vi "Start or Acquire.vi"(6 "Daq cmd":T2, 8 "error in (no error)":errorcluster) -> (0 "error out":errorcluster, 2 "Server Stats":T1={"scan rate"=10.0, "# connections"=0, "channel settings"=[]} {"channel settings"."lower input limits" format="%.4f"; "channel settings"."upper input limits" format="%.4f"; "scan rate" format="%.2f"}, 3 "task out":refnum<k21>)   [LabVIEW 2012]
uses:
  Local Daq Config.ctl
  Daq cmd.ctl
  DataServer/Server stats.ctl
  read-write.ctl
  ini interface.ctl
  <vilib>/DAQmx/read.llb/DAQmx Read (Analog 2D DBL NChan NSamp).vi
  <vilib>/DAQmx/create/channels.llb/DAQmx Create Channel (AI-Voltage-Basic).vi
  <vilib>/DAQmx/configure/timing.llb/DAQmx Timing (Sample Clock).vi
  <vilib>/DAQmx/miscellaneous.llb/DAQmx Fill In Error Info.vi
panel:
  out "data":dbl[][](array[numeric]) format="%0.2f"
  out "Channels":string
  in  "max buffer":i32=100
  out "Local Daq Config":T3={"Sample rate (Hz)"=1.0, "Over sample factor"=1.0, "Terminal Configuration"=enum."Single Ended", "Device"=0, "Max Voltage"=0} {"Device" items=["Dev1"]; "Over sample factor" min=1.0 max=125.0 step=1.0; "Sample rate (Hz)" min=1.0 max=10000.0 step=1.0}
  # "Hz"
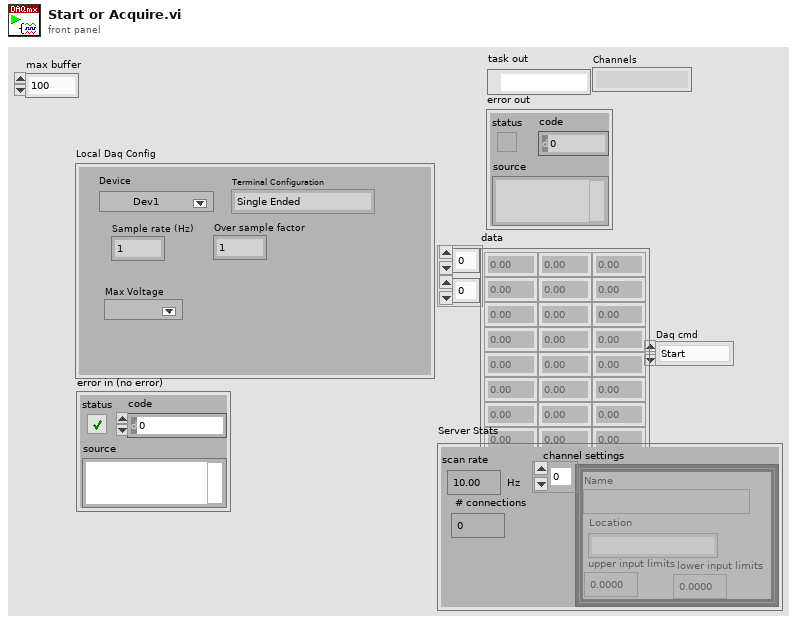
[diagram p1: front panel]
types:
  T1 = typedef "Server stats.ctl" = cluster{"scan rate":dbl, "# connections":i32, "channel settings":cluster{"Name":string, "upper input limits":sgl, "lower input limits":sgl, "Location":string}[]}
  T2 = typedef "Daq cmd.ctl" = enum16{"Start", "Get one scan", "Server Stats", "Stop Acquisition"}
  T3 = typedef "Local Daq Config.ctl" = cluster{"Sample rate (Hz)":dbl, "Over sample factor":dbl, "Terminal Configuration":enum16{"Single Ended", "Differential"}, "Device":u16, "Max Voltage":u16}
  T4 = typedef "ini interface.ctl" = enum16{"dataserver list", "dataserver", "com port", "stamp model", "Local Daq"}
  T5 = typedef "read-write.ctl" = enum16{"read", "write"}
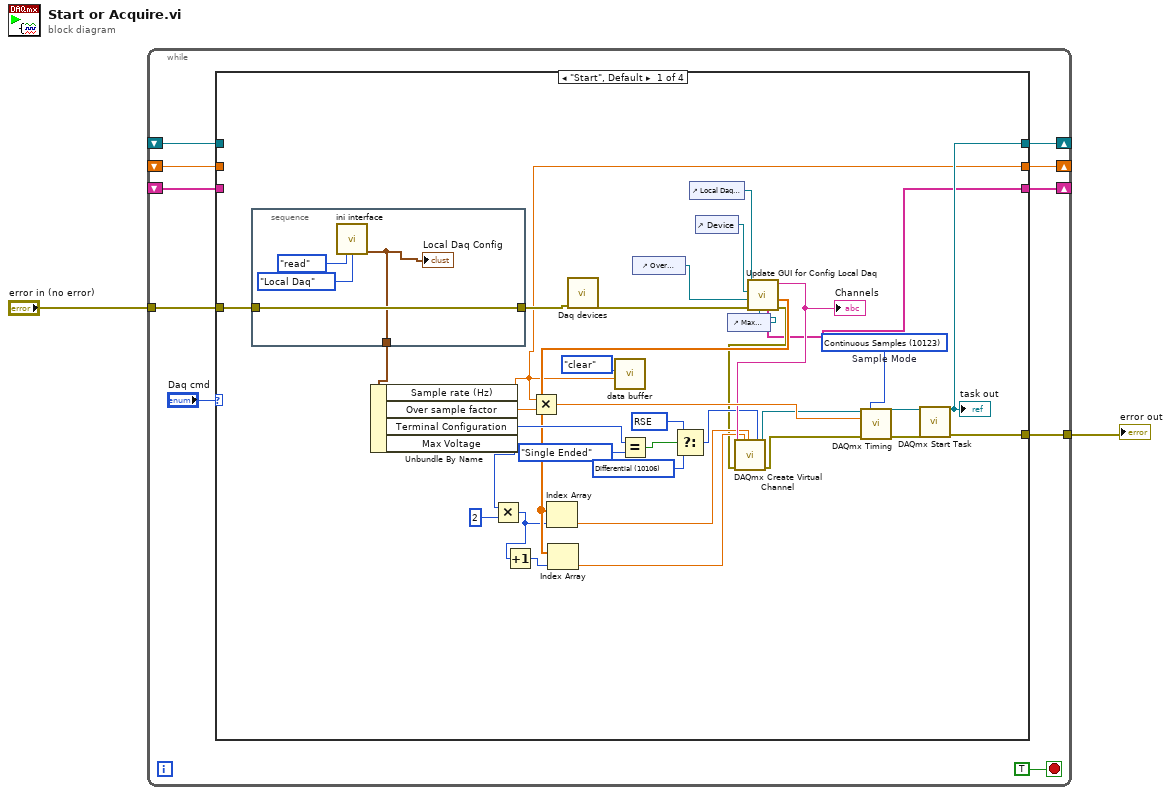
[diagram p0: block diagram]
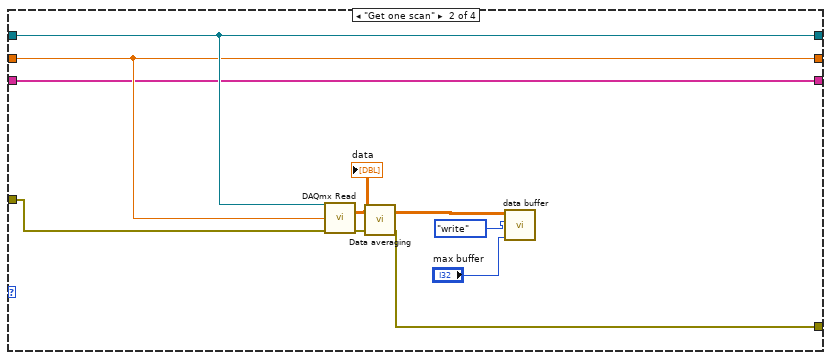
[diagram p2: hidden frame]
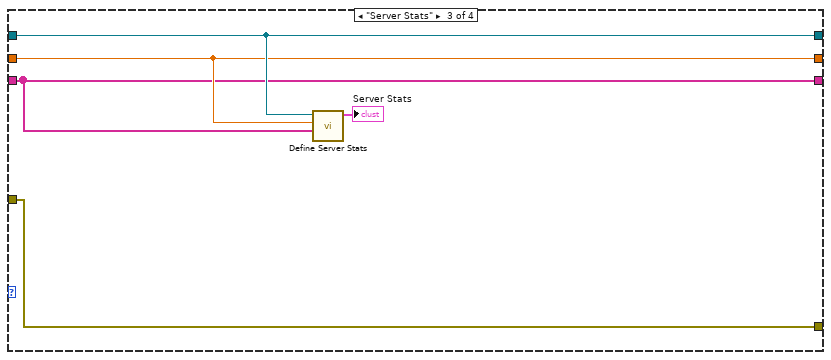
[diagram p3: hidden frame]
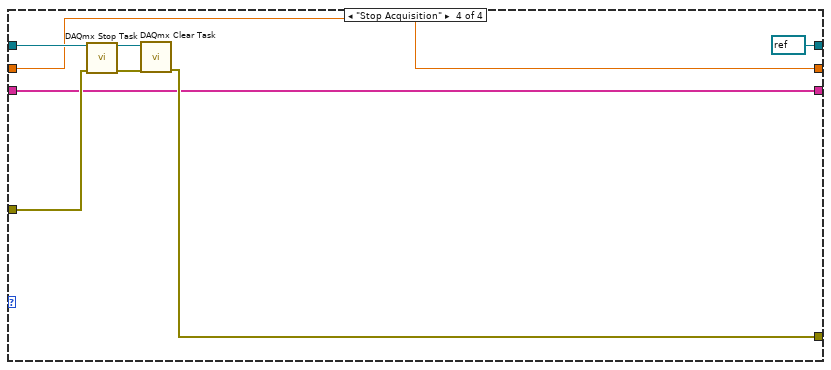
[diagram p4: hidden frame]
diagram:
  n1 = while {
    tunnel: [w12] -> w2
    tunnel: "error in (no error)" -> [w11]
    shift-right: [w9] -> _
    shift-left: _ -> [w8]
    shift-right: [w7] -> _
    shift-left: _ -> [w6]
    shift-right: [w4] -> _
    shift-left: _ -> [w3]
    stop <- TRUE stop-if-true
    n2 = case shown="\"Start\", Default" "Daq cmd" {
      tunnel: [w18 w55 w62 w69] -> w12
      tunnel: w11 -> [w16 w56 w62 w70]
      tunnel: [w15 w54 w65 refnum<k21> refnum ("task out")] -> w9
      tunnel: w8 -> [_ w54 w65 w73]
      tunnel: [w14 w53 w64 w67] -> w7
      tunnel: w6 -> [_ w53 w64 w67]
      tunnel: [w13 w52 w61 w66] -> w4
      tunnel: w3 -> [_ w52 w61 w66]
      frame "Start", Default {
        w20 = 10123 items=["Finite Samples"=10178, "Continuous Samples"=10123, "Hardware Timed Single Point"=12522]  # Sample Mode
        w34 = 10106 items=["default"=-1, "RSE"=10083, "NRSE"=10078, "Differential"=10106, "Pseudodifferential"=12529] ("input terminal configuration")
        w35 = 10083 items=["default"=-1, "RSE"=10083, "NRSE"=10078, "Differential"=10106, "Pseudodifferential"=12529] ("input terminal configuration")
        n3 = stacked-sequence {
          tunnel: w16 -> [w49]
          tunnel: [w49] -> w47
          tunnel: [w48] -> w45
          frame #0 {
            n4 = call "ini interface.vi"("direction"=read-write."read", "ini interface"=ini_interface."Local Daq") -> ("Local Daq Config out"=w48:T3)  [unwired: 9 in, 4 out]
            "Local Daq Config" <- w48
          }
        }
        n5 = Unbundle By Name(w45) -> ("Sample rate (Hz)"=w14:dbl, "Over sample factor"=w44:dbl, "Terminal Configuration"=w28:enum16{"Single Ended", "Differential"}, "Max Voltage"=w27:u16)
        n6 = Multiply(x=w27, y=u16 2) -> (x*y=w23:u16)
        n7 = Increment(x=w23) -> (x+1=w22:u16)
        n8 = Multiply(x=w14, y=w44) -> (x*y=w43:dbl)
        n9 = call "Daq devices.vi"("error in"=w47) -> ("error out"=w46:errorcluster)  [unwired: 5 in, 4 out]
        n10 = call "data buffer.vi"("action"=enum16{"write", "read", "clear"}."clear", "scan rate (Hz)"=w14) -> ()  [unwired: 2 in, 6 out]
        n11 = Equal?(x=w28, y=enum16{"Single Ended", "Differential"}."Single Ended") -> (x = y?=w36:bool)
        n12 = control-ref of="Over sample factor"() -> (w29:refnum<vi>)
        n13 = Select(t=w35, s=w36, f=w34) -> (s? t:f=w33:i32)
        n14 = control-ref of="Local Daq Config"() -> (w31:refnum<vi>)
        n15 = control-ref of="Device"() -> (w32:refnum<vi>)
        n16 = control-ref of="Max Voltage"() -> (w30:refnum<vi>)
        n17 = call "Update GUI for Config Local Daq.vi"("Voltage Ring"=w30, "error in (no error)"=w46, "Digital in"=w29, "Ring Refnum"=w32, "Clust Refnum 2"=w31) -> ("error out"=w19:errorcluster, "AI.Voltage.Rngs"=w25:dbl[], "Channels"=w38:string, "Port locations"=w13:string[])  [unwired: 2 in, 1 out]
        "Channels" <- w38
        n18 = Index Array(array=w25, index=w23) -> (element=w24:dbl)
        n19 = Index Array(array=w25, index=w22) -> (element=w21:dbl)
        n20 = call-poly <vilib>:"DAQmx Create Virtual Channel.vi"("maximum value"=w21, "minimum value"=w24, "input terminal configuration"=w33, "physical channels"=w38, "error in"=w19) -> ("task out"=w39:refnum<k21>, "error out"=w42:errorcluster)  [unwired: 9 in]
        n21 = call-poly <vilib>:"DAQmx Timing.vi"("task/channels in"=w39, "sample mode"=w20, "rate"=w43, "error in"=w42) -> ("task out"=w40:refnum<k21>, "error out"=w41:errorcluster)  [unwired: 10 in]
        n22 = call <vilib>:"DAQmx Start Task.vi"("task/channels in"=w40, "error in"=w41) -> ("task out"=w15:refnum<k21>, "error out"=w18:errorcluster)  [unwired: 12 in]
        "task out" <- w15
      }
      frame "Get one scan" {
        n23 = call-poly <vilib>:"DAQmx Read.vi"("task/channels in"=w54, "number of samples per channel"=w53, "error in"=w56) -> ("data"=w58:dbl[][], "error out"=w55:errorcluster)  [unwired: 10 in, 1 out]
        "data" <- w58
        n24 = call "Data averaging.vi"("data"=w58) -> ("Averaged data"=w59:dbl[][])  [unwired: 2 in]
        n25 = call "data buffer.vi"("voltage data"=w59, "action"=enum16{"write", "read", "clear"}."write", "max buffer"="max buffer") -> ()  [unwired: 1 in, 6 out]
      }
      frame "Server Stats" {
        n26 = call "Define Server Stats.vi"("Port locations"=w61, "scan rate (Hz)"=w64, "Refnum in"=w65) -> ("Server Stats"=→"Server Stats":T1)  [unwired: 6 in, 2 out]
      }
      frame "Stop Acquisition" {
        n27 = call <vilib>:"DAQmx Stop Task.vi"("task/channels in"=w73, "error in"=w70) -> ("task out"=w72:refnum<k21>, "error out"=w71:errorcluster)  [unwired: 12 in]
        n28 = call <vilib>:"DAQmx Clear Task.vi"("task in"=w72, "error in"=w71) -> ("error out"=w69:errorcluster)  [unwired: 13 in]
      }
    }
  }
  "error out" <- w2
